vi "62_Vision_RC Servo_c.vi"() -> ()   [LabVIEW 2018]
uses:
  <userlib>/KNR OS 4.0 LabVIEW Toolkit/Type Definition/Resource.ctl
  <userlib>/KNR OS 4.0 LabVIEW Toolkit/Type Definition/RC Servo Port.ctl
panel:
  out "RC Pulse Width (uS)":u16[](array[numeric])
  out "Image Out":T1(plugin-control)
  in  "stop":bool
  # "找不到目標停止servo"
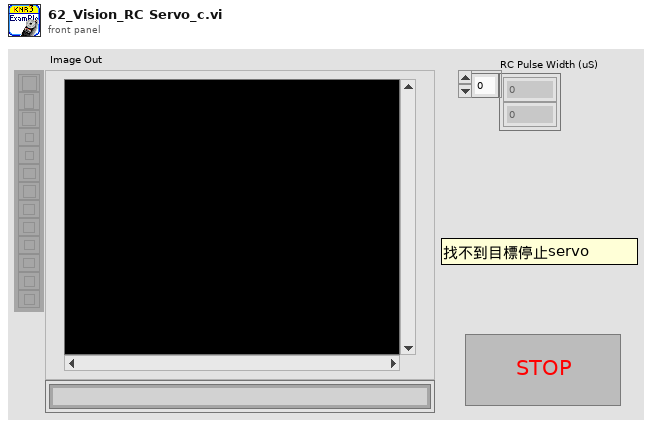
[diagram p1: front panel]
types:
  T1 = typedef "IMAQ Image.ctl" = refnum<image>
  T2 = typedef "RC Servo Port.ctl" = u16
  T3 = typedef "Resource.ctl" = enum16{"KNRm_DDRC", "KNRm_DDDD", "KNRm_DDDR", "KNRm_DDDC", "KNR", "KNRm_neww"}
  T4 = typedef "KNR3 Reference.ctl" = cluster{"FPGA Session":refnum<class "FPGA Interface Base.lvclass">, "Resource":T3}
  T5 = cluster{"Left":dbl, "Top":dbl, "Right":dbl, "Bottom":dbl}
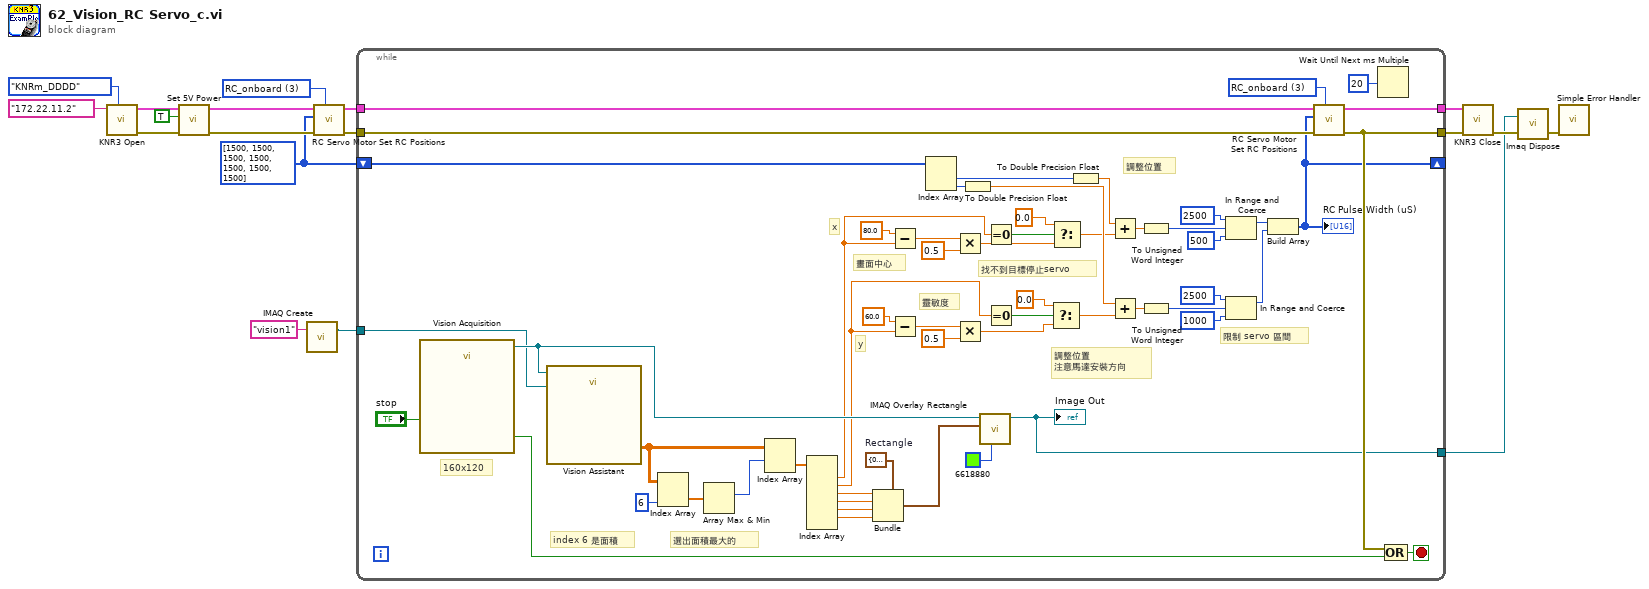
[diagram p0: block diagram]
diagram:
  w4 = u16[] [1500, 1500, 1500, 1500, 1500, 1500, 1500] ("RC Pulse Width (1500 uS)")
  w7 = T2 3 items=["RC_onboard"=3, "RC_box"=9] ("Port (RC_onboard)")
  n1 = call <userlib>:"KNR3 Open.vi"("Resource"=Resource."KNRm_DDDD", "IP"="172.22.11.2") -> ("error out"=w15:errorcluster, "KNR out"=w17:T4)  [unwired: 8 in]
  n2 = call <userlib>:"Set 5V Power.vi"("error in (no error)"=w15, "5V Power(T)"=TRUE ("5V Power"), "KNR in"=w17) -> ("error out"=w14:errorcluster, "KNR out"=w16:T4)  [unwired: 7 in]
  n3 = call "IMAQ Create"("Image Name"="vision1") -> ("New Image"=w5:T1)  [unwired: 4 in, 1 out]
  n4 = call <userlib>:"RC Servo Motor Set RC Positions.vi"("Port (RC_onboard)"=w7, "RC Pulse Width (1500 uS)"=w4, "KNR in"=w16) -> ("KNR out"=w8:T4)  [unwired: 7 in, 1 out]
  n5 = while {
    tunnel: w8 -> [w73]
    tunnel: [w72] -> w10
    tunnel: w14 -> [w71]
    tunnel: [w69] -> w9
    tunnel: w5 -> [w53]
    shift-right: [w35] -> _
    shift-left: w4 -> [w38]
    tunnel: [w18] -> w1
    stop <- w70 stop-if-true
    w65 = T5 {"Left"=0.0, "Top"=0.0, "Right"=0.0, "Bottom"=0.0}  # Rectangle
    w67 = T2 3 items=["RC_onboard"=3, "RC_box"=9] ("RC Motor")
    # "調整位置\n注意馬達安裝方向"
    # "index 6 是面積"
    # "調整位置"
    # "限制 servo 區間"
    # "靈敏度"
    # "畫面中心"
    # "找不到目標停止servo"
    # "y"
    # "x"
    # "160x120"
    # "選出面積最大的"
    n6 = call "Vision Acquisition"("Stop (F)"="stop") -> ("Image Out"=w58:T1, "Stopped"=w51:bool)  [unwired: 24 in, 1 out]
    n7 = call "Vision Assistant"("Image In"=w58, "Image Dst"=w53) -> ("Particle Measurements (Pixels) (Particle Analysis 1)"=w57:dbl[][])  [unwired: 22 in, 3 out]
    n8 = Index Array "Index Array"(array=w57, index (col)=6 ("disabled index (col)")) -> (element=w56:dbl[])  [unwired: 1 in]
    n9 = Array Max & Min(array=w56) -> (max index (indices)=w55:i32)  [unwired: 3 out]
    n10 = Index Array "Index Array"(array=w57, index (row)=w55) -> (element=w66:dbl[])  [unwired: 1 in]
    n11 = Index Array "Index Array"(array=w66) -> (element #1=w27:dbl, element #2=w19:dbl, element #3=w64:dbl, element #4=w63:dbl, element #5=w62:dbl, element #6=w61:dbl)  [unwired: 7 in, 1 out]
    n12 = Bundle "Bundle"(cluster=w65, "Left"=w64, "Top"=w63, "Right"=w62, "Bottom"=w61) -> (w60:T5)
    n13 = Subtract(x=80.0 ("y"), y=w27) -> (x-y=w47:dbl)
    n14 = Subtract(x=60.0 ("y"), y=w19) -> (x-y=w48:dbl)
    n15 = Index Array "Index Array"(array=w38) -> (element #1=w37:u16, element #2=w36:u16)  [unwired: 2 in]
    n16 = Multiply(x=w47, y=0.5) -> (x*y=w25:dbl)
    n17 = Multiply(x=w48, y=0.5) -> (x*y=w21:dbl)
    n18 = To Double Precision Float(number=w36) -> (double precision float=w29:dbl)
    n19 = call "IMAQ Overlay Rectangle"("Color"=u32 6618880, "Rectangle"=w60, "Image"=w58) -> ("Image Out"=w18:T1)  [unwired: 7 in, 1 out]
    "Image Out" <- w18
    n20 = Equal To 0?(x=w27) -> (x = 0?=w28:bool)
    n21 = Equal To 0?(x=w19) -> (x = 0?=w22:bool)
    n22 = Select(t=0.0, s=w22, f=w21) -> (s? t:f=w20:dbl)
    n23 = Select(t=0.0, s=w28, f=w25) -> (s? t:f=w24:dbl)
    n24 = To Double Precision Float(number=w37) -> (double precision float=w30:dbl)
    n25 = Add(x=w30, y=w24) -> (x+y=w49:dbl)
    n26 = Add(x=w29, y=w20) -> (x+y=w50:dbl)
    n27 = To Unsigned Word Integer(number=w49) -> (unsigned 16bit integer=w32:u16)
    n28 = To Unsigned Word Integer(number=w50) -> (unsigned 16bit integer=w31:u16)
    n29 = In Range and Coerce(upper limit=u16 2500, x=w32, lower limit=u16 500) -> (coerced(x)=w45:u16)  [unwired: 1 out]
    n30 = In Range and Coerce(upper limit=u16 2500, x=w31, lower limit=u16 1000) -> (coerced(x)=w46:u16)  [unwired: 1 out]
    n31 = Build Array(w45, w46) -> (w35:u16[])
    "RC Pulse Width (uS)" <- w35
    n32 = call <userlib>:"RC Servo Motor Set RC Positions.vi"("Port (RC_onboard)"=w67, "error in (no error)"=w71, "RC Pulse Width (1500 uS)"=w35, "KNR in"=w73) -> ("error out"=w69:errorcluster, "KNR out"=w72:T4)  [unwired: 6 in]
    n33 = Wait Until Next ms Multiple(millisecond multiple=u32 20) -> ()  [unwired: 1 out]
    n34 = Compound Arithmetic op=OR(w69, w51) -> (w70:bool)
  }
  n35 = call <userlib>:"KNR3 Close.vi"("error in (no error)"=w9, "KNR in"=w10) -> ("error out"=w3:errorcluster)  [unwired: 9 in]
  n36 = call "Imaq Dispose"("Image"=w1, "error in (no error)"=w3) -> ("error out"=w2:errorcluster)  [unwired: 4 in]
  n37 = call <vilib>:"Simple Error Handler.vi"("error in (no error)"=w2) -> ()  [unwired: 4 in, 5 out]
